vi "Close.vi"(8 "error in":errorcluster) -> (0 "error out":errorcluster)   [LabVIEW 2014]
doc: "This function closes the serial connection to the device and should be used every time testing stops for half hour or more."
uses:
  Private/Controls/Global Megger.vi
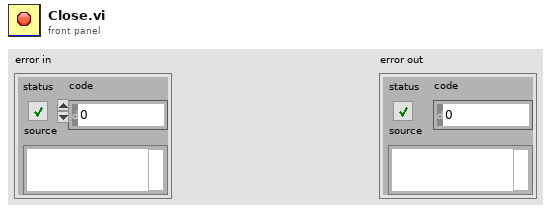
[diagram p1: front panel]
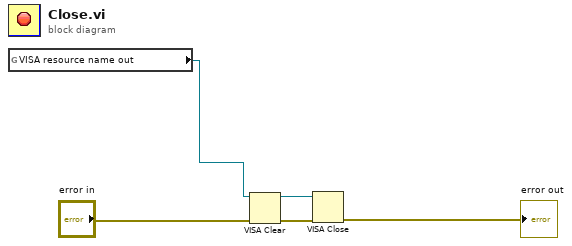
[diagram p0: block diagram]
diagram:
  n1 = global read "Global Megger.vi" "VISA resource name out"() -> (w3:refnum<visa-resource-name>)
  n2 = VISA Clear(VISA resource name=w3, error in (no error)="error in") -> (VISA resource name out=w1:refnum<visa-resource-name>, error out=w4:errorcluster)
  n3 = VISA Close(VISA resource name=w1, error in (no error)=w4) -> (error out=→"error out":errorcluster)
